vi "最大值最小值.vi"(2 "reset":bool, 3 "Input":dbl) -> (0 "MIN":dbl, 1 "MAX":dbl)   [LabVIEW 2018]
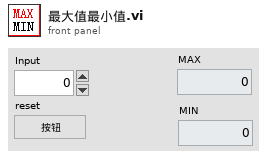
[diagram p1: front panel]
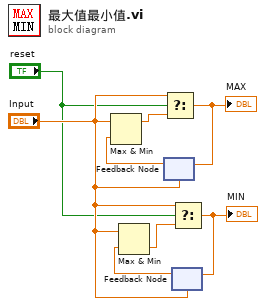
[diagram p0: block diagram]
diagram:
  n1 = feedback #1("Input") -> (w7:dbl)
  n2 = Max & Min(x="Input", y=w7) -> (max(x,y)=w8:dbl)  [unwired: 1 out]
  n3 = Select(t="Input", s="reset", f=w8) -> (s? t:f=w6:dbl)
  "MAX" <- w6
  n4 = feedback-in #1(w6) -> ()
  n5 = feedback #2("Input") -> (w5:dbl)
  n6 = Max & Min(x="Input", y=w5) -> (min(x,y)=w4:dbl)  [unwired: 1 out]
  n7 = Select(t="Input", s="reset", f=w4) -> (s? t:f=w1:dbl)
  "MIN" <- w1
  n8 = feedback-in #2(w1) -> ()
